vi "Car Wash.vi"() -> ()   [LabVIEW 2023]
uses:
  Controls/Car Wash Indicators.ctl
  Controls/Wash Options.ctl
  Controls/Queued_Data.ctl
  Controls/State.ctl
  Controls/System_Data.ctl
panel:
  out "error out":errorcluster
  in  "error in":errorcluster
  in  "Start":bool
  out "Elapsed Time":dbl format="%0.2f"
  in  "stop":bool
  out "Wash Entry":bool
  in  "Wash Options":T1
  in  "Car Position Slider":u8(slide) max=3 scale=0.0..4.0
  out "Car Wash Indicators":T2
  # "Car Wash Display"
  # "Entry Console"
  # "Car Position Simulation"
  # "Pre-Soak\nH-P Wash\nL-P Wax\nSpot Free Rinse"
  # "Underbody Wash\nBug Remover"
  # "Tire Shine\nAir Dry"
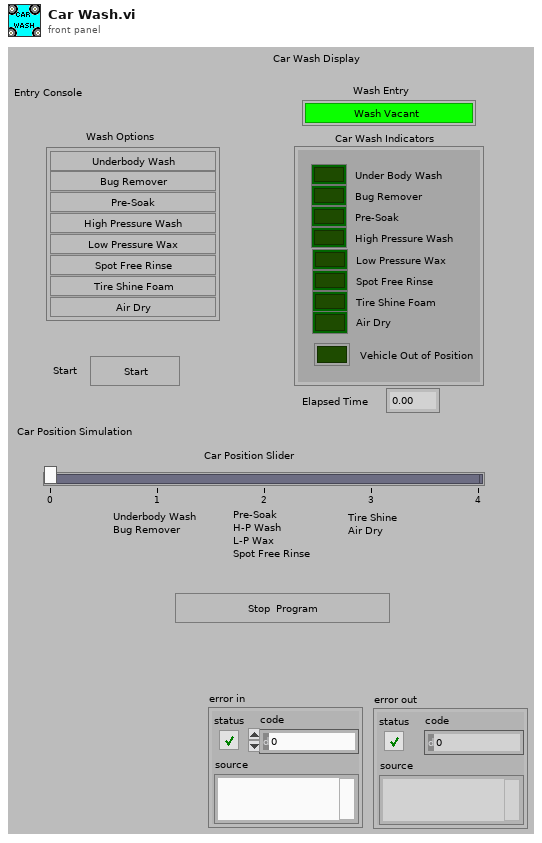
[diagram p1: front panel]
types:
  T1 = typedef "Wash Options.ctl" = cluster{"Underbody Wash":bool, "Bug Remover":bool, "Pre-Soak":bool, "High Pressure Wash":bool, "Low Pressure Wax":bool, "Spot Free Rinse":bool, "Tire Shine Foam":bool, "Air Dry":bool}
  T2 = typedef "Car Wash Indicators.ctl" = cluster{"Under Body Wash":bool, "Bug Remover":bool, "Pre-Soak":bool, "High Pressure Wash":bool, "Low Pressure Wax":bool, "Spot Free Rinse":bool, "Tire Shine Foam":bool, "Air Dry":bool, "Vehicle Out of Position":bool}
  T3 = typedef "State.ctl" = enum16{"Initialize", "Wait for Something", "Step Completed", "Save Wash Options", "Start Process", "Car Position", "Order Steps to follow", "Underbody Wash", "Bug Remover", "Pre-Soak", "High Pressure Wash", "Low Pressure Wax", "Spot Free Rinse", "Tire Shine Foam", "Air Dry", "Vehicle out of position", "Process Complete", "Stop Application"}
  T4 = enum8{"Enabled", "Disabled", "Disabled and Grayed Out"}
  T5 = typedef "System_Data.ctl" = cluster{"Start button":bool, "Wash Options":T1, "Enabled Steps Index":i32[], "Enabled Steps ":T3[], "Index Current Step":i32, "Car Position":u8, "Step Time":dbl[], "Timeout":i32}
  T6 = typedef "Queued_Data.ctl" = cluster{"State":T3, "Data":variant}
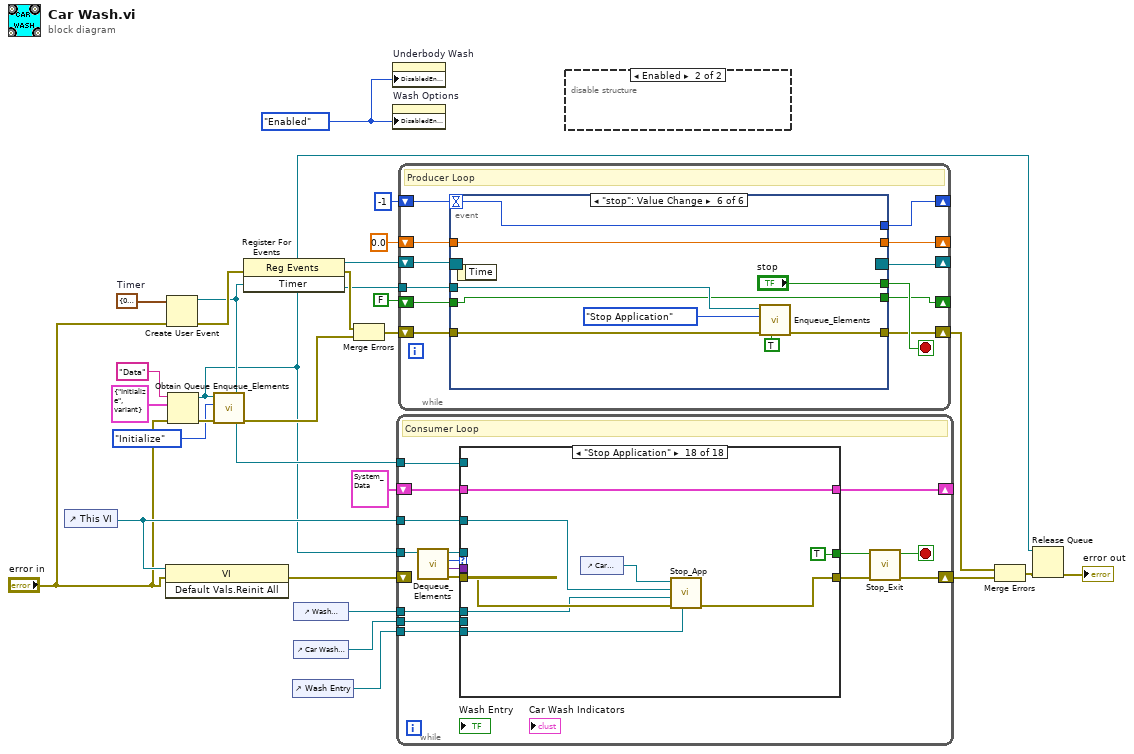
[diagram p0: block diagram]
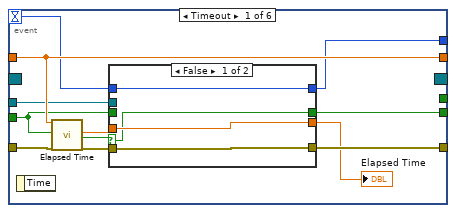
[diagram p2: hidden frame]
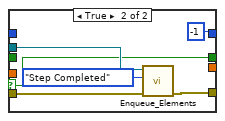
[diagram p3: hidden frame]
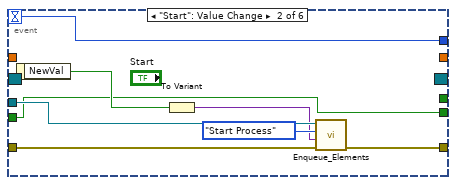
[diagram p4: hidden frame]
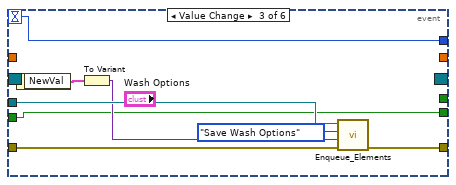
[diagram p5: hidden frame]
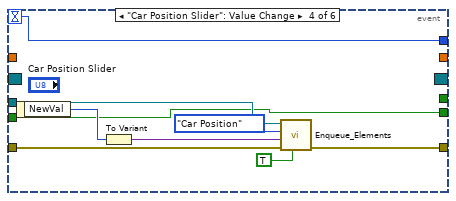
[diagram p6: hidden frame]
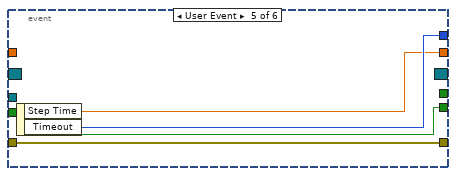
[diagram p7: hidden frame]
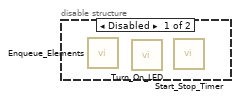
[diagram p8: hidden frame]
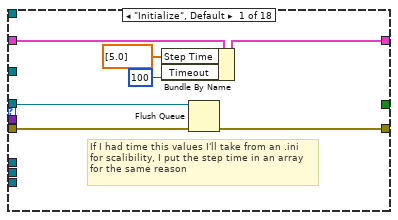
[diagram p9: hidden frame]
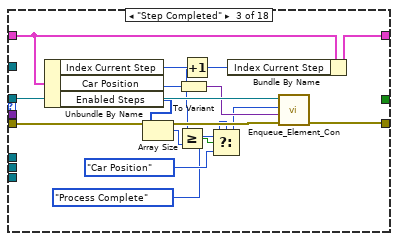
[diagram p11: hidden frame]
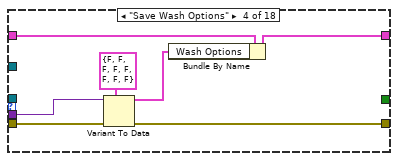
[diagram p12: hidden frame]
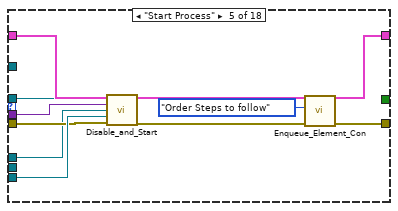
[diagram p13: hidden frame]
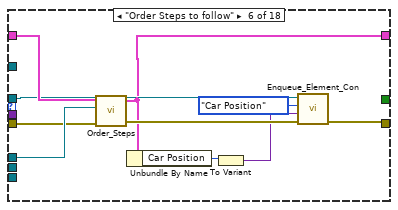
[diagram p14: hidden frame]
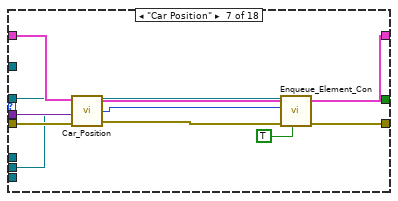
[diagram p15: hidden frame]
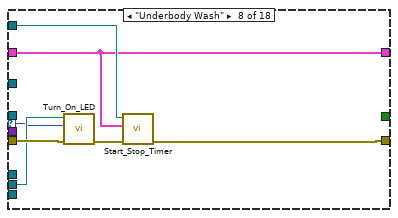
[diagram p16: hidden frame]
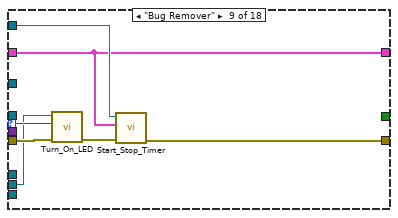
[diagram p17: hidden frame]
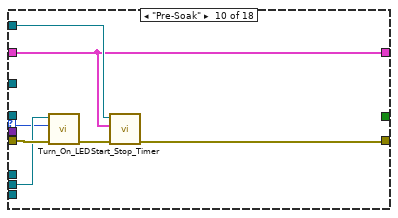
[diagram p18: hidden frame]
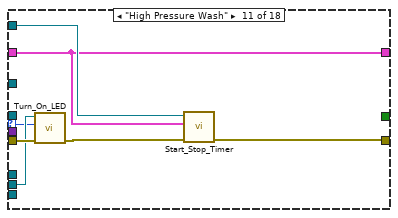
[diagram p19: hidden frame]
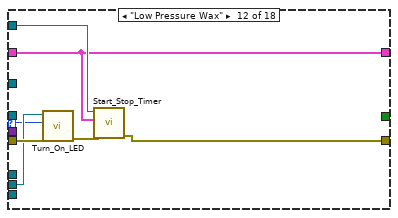
[diagram p20: hidden frame]
diagram:
  w8 = cluster{"Step Time":dbl, "Timeout":i32} {"Step Time"=0.0, "Timeout"=0}  # Timer
  w19 = T4."Enabled" ("Disabled")
  n1 = control-ref of="This VI"() -> (w18:refnum<vi>)
  n2 = invoke class="VI" method="Default Vals.Reinit All"(reference=w18, error in="error in") -> (error out=w17:errorcluster)  [unwired: 1 in, 2 out]
  n3 = Create User Event(user event datatype=w8, error in="error in") -> (user event=w10:refnum<user-event>, error out=w12:errorcluster)
  n4 = Obtain Queue(name (unnamed)="Data", element data type=T6 {"State"=enum."Initialize", "Data"=variant}, error in (no error)="error in") -> (queue out=w2:refnum<queue>, error out=w5:errorcluster)  [unwired: 2 in, 1 out]
  n5 = call "Enqueue_Elements.vi"("error in (no error)"=w5, "State"=State."Initialize", "Queue in"=w2) -> ("error out"=w4:errorcluster)  [unwired: 8 in]
  n6 = register-events(error in=w12, w10) -> (reference out=w11:refnum<event-registration>, error out=w13:errorcluster)  [unwired: 1 in]
  n7 = control-ref of="Wash Entry"() -> (w21:refnum<vi>)
  n8 = control-ref of="Wash Options"() -> (w20:refnum<vi>)
  n9 = control-ref of="Car Wash Indicators"() -> (w22:refnum<vi>)
  n10 = Merge Errors(w13, w4) -> (w15:errorcluster)
  n11 = property on="Underbody Wash" class="Bool (strict)"("DisabledEnum"=w19) -> ()  [unwired: 2 in, 2 out]
  n12 = property on="Wash Options" class="Clust (strict)"("DisabledEnum"=w19) -> ()  [unwired: 2 in, 2 out]
  n13 = while {
    shift-right: [w41] -> w26
    shift-left: w17 -> [_]
    tunnel: w2 -> [w39]
    shift-right: [w36] -> _
    shift-left: T5 {"Start button"=FALSE, "Wash Options"={"Underbody Wash"=FALSE, "Bug Remover"=FALSE, "Pre-Soak"=FALSE, "High Pressure Wash"=FALSE, "Low Pressure Wax"=FALSE, "Spot Free Rinse"=FALSE, "Tire Shine Foam"=FALSE, "Air Dry"=FALSE}, "Enabled Steps Index"=[], "Enabled Steps "=[], "Index Current Step"=0, "Car Position"=0, "Step Time"=[], "Timeout"=0} -> [w37]
    tunnel: w20 -> [w34]
    tunnel: w22 -> [w30]
    tunnel: w21 -> [w33]
    tunnel: w18 -> [w32]
    tunnel: w10 -> [w28]
    stop <- w43 stop-if-true
    # "Consumer Loop"
    n14 = call "Dequeue_Elements.vi"("Queue in"=w39) -> ("error out"=w40:errorcluster, "Data"=w38:variant, "State"=w29:T3, "queue out"=w35:refnum<queue>)  [unwired: 3 in]
    n15 = case shown="\"Stop Application\"" w29 {
      selector: w29 -> [_ _ _ _ _ _ _ w109 w118 w123 w130 w137 w144 w151 w158 _ _ _]
      tunnel: w40 -> [w50 w52 w64 w74 w77 w92 w104 w111 w117 w125 w132 w139 w146 w153 w160 w170 w172 w179]
      tunnel: [w45 w52 w63 w72 w75 w90 w100 w107 w114 w121 w128 w135 w142 w148 w156 w166 w173 w181] -> w42
      tunnel: w38 -> [_ _ _ w71 w83 _ w102 _ _ _ _ _ _ _ _ _ _ _]
      tunnel: w37 -> [w49 w51 w67 w73 w84 w94 w103 w105 w112 w119 w126 w133 w140 w147 w154 w169 w174 w182]
      tunnel: [w48 w51 w65 w69 w82 w87 w101 w105 w112 w119 w126 w133 w140 w147 w154 w169 w174 w182] -> w36
      tunnel: w35 -> [w44 _ w62 _ w80 w89 w98 _ _ _ _ _ _ _ _ _ _ _]
      tunnel: w34 -> [_ _ _ _ w76 w93 _ _ _ _ _ _ _ _ _ _ _ w178]
      tunnel: w30 -> [_ _ _ _ _ _ w95 w110 w116 w124 w131 w138 w145 w152 w159 w167 _ _]
      tunnel: w33 -> [_ _ _ _ w78 _ _ _ _ _ _ _ _ _ _ _ _ w176]
      tunnel: w32 -> [_ _ _ _ _ _ _ _ _ _ _ _ _ _ _ _ w171 w180]
      tunnel: [_ _ _ _ _ _ _ _ _ _ _ _ _ _ _ _ _ TRUE] -> w31
      tunnel: w28 -> [_ _ _ _ _ _ _ w106 w113 w120 w127 w134 w141 w149 w155 _ _ _]
      frame "Initialize", Default {
        # "If I had time this values I'll take from an .ini\nfor scalibility, I put the step time in an array\nfor the same reason"
        n16 = Bundle By Name(cluster=w49, "Step Time"=dbl[] [5.0], "Timeout"=100) -> (w48:T5)
        n17 = Flush Queue(queue=w44, error in (no error)=w50) -> (error out=w45:errorcluster)  [unwired: 2 out]
      }
      frame "Wait for Something" {
      }
      frame "Step Completed" {
        n18 = Unbundle By Name(w67) -> ("Index Current Step"=w66:i32, "Car Position"=w61:u8, "Enabled Steps"=w58:T3[])
        n19 = Array Size(array=w58) -> (size(s)=w57:i32)
        n20 = To Variant(anything=w61) -> (Variant=w60:variant)
        n21 = Increment(x=w66) -> (x+1=w59:i32)
        n22 = Greater Or Equal?(x=w59, y=w57) -> (x >= y?=w56:bool)
        n23 = Select(t=State."Process Complete" ("State"), s=w56, f=State."Car Position" ("State")) -> (s? t:f=w54:T3)
        n24 = Bundle By Name(cluster=w67, "Index Current Step"=w59) -> (w65:T5)
        n25 = call "Enqueue_Element_Con.vi"("error in (no error)"=w64, "Data"=w60, "State"=w54, "Queue in"=w62) -> ("error out"=w63:errorcluster)  [unwired: 7 in]
      }
      frame "Save Wash Options" {
        n26 = Variant To Data(error in=w74, type=T1 {"Underbody Wash"=FALSE, "Bug Remover"=FALSE, "Pre-Soak"=FALSE, "High Pressure Wash"=FALSE, "Low Pressure Wax"=FALSE, "Spot Free Rinse"=FALSE, "Tire Shine Foam"=FALSE, "Air Dry"=FALSE} ("Wash Options"), Variant=w71) -> (data=w68:T1, error out=w72:errorcluster)
        n27 = Bundle By Name(cluster=w73, "Wash Options"=w68) -> (w69:T5)
      }
      frame "Start Process" {
        n28 = call "Disable_and_Start.vi"("System data in"=w84, "Data"=w83, "Wash Options In"=w76, "Wash Entry"=w78, "error in (no error)"=w77) -> ("System data out"=w82:T5, "error out"=w81:errorcluster)  [unwired: 9 in]
        n29 = call "Enqueue_Element_Con.vi"("error in (no error)"=w81, "State"=State."Order Steps to follow", "Queue in"=w80) -> ("error out"=w75:errorcluster)  [unwired: 8 in]
      }
      frame "Order Steps to follow" {
        n30 = call "Order_Steps.vi"("System data"=w94, "Wash Options"=w93, "error in (no error)"=w92) -> ("System data out"=w87:T5, "error out"=w91:errorcluster)  [unwired: 3 in]
        n31 = Unbundle By Name(w87) -> ("Car Position"=w86:u8)
        n32 = To Variant(anything=w86) -> (Variant=w85:variant)
        n33 = call "Enqueue_Element_Con.vi"("error in (no error)"=w91, "Data"=w85, "State"=State."Car Position", "Queue in"=w89) -> ("error out"=w90:errorcluster)  [unwired: 7 in]
      }
      frame "Car Position" {
        n34 = call "Car_Position.vi"("error in (no error)"=w104, "Car Wash Indicators"=w95, "Data"=w102, "System data in"=w103) -> ("error out"=w99:errorcluster, "State"=w97:T3, "System data out"=w101:T5)
        n35 = call "Enqueue_Element_Con.vi"("Prioritize?"=TRUE, "error in (no error)"=w99, "State"=w97, "Queue in"=w98) -> ("error out"=w100:errorcluster)  [unwired: 7 in]
      }
      frame "Underbody Wash" {
        n36 = call "Turn_On_LED.vi"("error in (no error)"=w111, "State"=w109, "Car Wash Indicators"=w110) -> ("error out"=w108:errorcluster)  [unwired: 8 in]
        n37 = call "Start_Stop_Timer.vi"("error in (no error)"=w108, "System data"=w105, "User Event in"=w106) -> ("error out"=w107:errorcluster)  [unwired: 8 in]
      }
      frame "Bug Remover" {
        n38 = call "Turn_On_LED.vi"("error in (no error)"=w117, "State"=w118, "Car Wash Indicators"=w116) -> ("error out"=w115:errorcluster)  [unwired: 8 in]
        n39 = call "Start_Stop_Timer.vi"("error in (no error)"=w115, "System data"=w112, "User Event in"=w113) -> ("error out"=w114:errorcluster)  [unwired: 8 in]
      }
      frame "Pre-Soak" {
        n40 = call "Turn_On_LED.vi"("error in (no error)"=w125, "State"=w123, "Car Wash Indicators"=w124) -> ("error out"=w122:errorcluster)  [unwired: 8 in]
        n41 = call "Start_Stop_Timer.vi"("error in (no error)"=w122, "System data"=w119, "User Event in"=w120) -> ("error out"=w121:errorcluster)  [unwired: 8 in]
      }
      frame "High Pressure Wash" {
        n42 = call "Turn_On_LED.vi"("error in (no error)"=w132, "State"=w130, "Car Wash Indicators"=w131) -> ("error out"=w129:errorcluster)  [unwired: 8 in]
        n43 = call "Start_Stop_Timer.vi"("error in (no error)"=w129, "System data"=w126, "User Event in"=w127) -> ("error out"=w128:errorcluster)  [unwired: 8 in]
      }
      frame "Low Pressure Wax" {
        n44 = call "Turn_On_LED.vi"("error in (no error)"=w139, "State"=w137, "Car Wash Indicators"=w138) -> ("error out"=w136:errorcluster)  [unwired: 8 in]
        n45 = call "Start_Stop_Timer.vi"("error in (no error)"=w136, "System data"=w133, "User Event in"=w134) -> ("error out"=w135:errorcluster)  [unwired: 8 in]
      }
      frame "Spot Free Rinse" {
        n46 = call "Turn_On_LED.vi"("error in (no error)"=w146, "State"=w144, "Car Wash Indicators"=w145) -> ("error out"=w143:errorcluster)  [unwired: 8 in]
        n47 = call "Start_Stop_Timer.vi"("error in (no error)"=w143, "System data"=w140, "User Event in"=w141) -> ("error out"=w142:errorcluster)  [unwired: 8 in]
      }
      frame "Tire Shine Foam" {
        n48 = call "Turn_On_LED.vi"("error in (no error)"=w153, "State"=w151, "Car Wash Indicators"=w152) -> ("error out"=w150:errorcluster)  [unwired: 8 in]
        n49 = call "Start_Stop_Timer.vi"("error in (no error)"=w150, "System data"=w147, "User Event in"=w149) -> ("error out"=w148:errorcluster)  [unwired: 8 in]
      }
      frame "Air Dry" {
        n50 = call "Turn_On_LED.vi"("error in (no error)"=w160, "State"=w158, "Car Wash Indicators"=w159) -> ("error out"=w157:errorcluster)  [unwired: 8 in]
        n51 = call "Start_Stop_Timer.vi"("error in (no error)"=w157, "System data"=w154, "User Event in"=w155) -> ("error out"=w156:errorcluster)  [unwired: 8 in]
      }
      frame "Vehicle out of position" {
        w162 = TRUE ("Vehicle Out of Position")
        n52 = property class="Clust (strict)"(reference=w167, error in=w170) -> (reference out=w165:refnum<vi>, error out=w168:errorcluster, "Value"=w164:T2)
        n53 = Not(x=w162) -> (.not. x?=w161:bool)
        n54 = Bundle By Name(cluster=w164, "Vehicle Out of Position"=w162, "Air Dry"=w161, "Tire Shine Foam"=w161, "Spot Free Rinse"=w161, "Low Pressure Wax"=w161, "High Pressure Wash"=w161, "Pre-Soak"=w161, "Bug Remover"=w161, "Under Body Wash"=w161) -> (w163:T2)
        n55 = property class="Clust (strict)"(reference=w165, error in=w168, "Value"=w163) -> (error out=w166:errorcluster)  [unwired: 1 out]
      }
      frame "Process Complete" {
        n56 = invoke class="VI" method="Default Vals.Reinit All"(reference=w171, error in=w172) -> (error out=w173:errorcluster)  [unwired: 1 in, 2 out]
      }
      frame "Stop Application" {
        n57 = control-ref of="Car Position"() -> (w177:refnum<vi>)
        n58 = call "Stop_App.vi"("Wash Entry"=w176, "error in (no error)"=w179, "Wash Options"=w178, "This VI"=w180, "Car Position"=w177) -> ("error out"=w181:errorcluster)  [unwired: 6 in]
      }
    }
    n59 = call "Stop_Exit.vi"("error in (no error)"=w42, "STOP button"=w31) -> ("error out"=w41:errorcluster, "Exit While"=w43:bool)  [unwired: 8 in]
  }
  n60 = while {
    tunnel: w2 -> [w194]
    shift-right: [w191] -> w14
    shift-left: w15 -> [w193]
    shift-right: [w189] -> _
    shift-left: w11 -> [w190]
    shift-right: [w187] -> _
    shift-left: -1 -> [w188]
    shift-right: [w185] -> _
    shift-left: 0.0 -> [w186]
    shift-right: [w183] -> _
    shift-left: FALSE -> [w184]
    stop <- w192 stop-if-true
    # "Producer Loop"
    n61 = event shown="[5] \"stop\": Value Change" {
      selector: w190 -> [_ _ _ _ _ _]
      dyn-events: [_ _ _ _ _ _] -> w189
      timeout: w188 -> [w202 w218 w226 w234 _ w248]
      tunnel: w194 -> [w197 w224 w230 w241 _ w253]
      tunnel: w193 -> [w206 w223 w231 w237 w245 w251]
      tunnel: [w200 w222 w232 w239 w245 w254] -> w191
      tunnel: [_ _ _ _ _ "stop"] -> w192
      tunnel: [w203 w218 w226 w234 w244 w248] -> w187
      tunnel: w186 -> [w205 _ _ _ _ w247]
      tunnel: [w205 _ _ _ w243 w247] -> w185
      tunnel: w184 -> [w196 w217 w225 w233 w242 w246]
      tunnel: [w195 w217 w225 w233 w242 w246] -> w183
      event Timeout {
        n62 = event-data() -> ()  [unwired: 1 in, 1 out]
        n63 = call "Elapsed Time"("Time Target (s)"=w205, "Reset"=w196, "error in (no error)"=w206) -> ("Elapsed Time (s)"=w198:dbl, "Time has Elapsed"=w204:bool, "error out"=w201:errorcluster)  [unwired: 9 in, 5 out]
        n64 = case shown="False" w204 {
          selector: w204 -> [w207 w211]
          tunnel: [w210 -1 ("t")] -> w203
          tunnel: w202 -> [w210 _]
          tunnel: w198 -> [w208 _]
          tunnel: w201 -> [w209 w214]
          tunnel: [w209 w215] -> w200
          tunnel: [w208 _] -> w199
          tunnel: w197 -> [_ w213]
          tunnel: w196 -> [_ _]
          tunnel: [w207 w211] -> w195
          frame False {
          }
          frame True {
            n65 = call "Enqueue_Elements.vi"("error in (no error)"=w214, "State"=State."Step Completed", "Queue in"=w213) -> ("error out"=w215:errorcluster)  [unwired: 8 in]
          }
        }
        "Elapsed Time" <- w199
      }
      event "Start": Value Change {
        n66 = event-data() -> ("NewVal"=w220:bool)  [unwired: 1 in]
        n67 = To Variant(anything=w220) -> (Variant=w219:variant)
        n68 = call "Enqueue_Elements.vi"("error in (no error)"=w223, "Data"=w219, "State"=State."Start Process", "Queue in"=w224) -> ("error out"=w222:errorcluster)  [unwired: 7 in]
      }
      event Value Change {
        n69 = event-data() -> ("NewVal"=w229:T1)  [unwired: 1 in]
        n70 = To Variant(anything=w229) -> (Variant=w227:variant)
        n71 = call "Enqueue_Elements.vi"("error in (no error)"=w231, "Data"=w227, "State"=State."Save Wash Options", "Queue in"=w230) -> ("error out"=w232:errorcluster)  [unwired: 7 in]
      }
      event "Car Position Slider": Value Change {
        n72 = event-data() -> ("NewVal"=w240:u8)  [unwired: 1 in]
        n73 = To Variant(anything=w240) -> (Variant=w236:variant)
        n74 = call "Enqueue_Elements.vi"("Prioritize?"=TRUE, "error in (no error)"=w237, "Data"=w236, "State"=State."Car Position", "Queue in"=w241) -> ("error out"=w239:errorcluster)  [unwired: 6 in]
      }
      event User Event {
        n75 = event-data() -> ("Step Time"=w243:dbl, "Timeout"=w244:i32)  [unwired: 1 in]
      }
      event "stop": Value Change {
        n76 = event-data() -> ()  [unwired: 1 in, 1 out]
        n77 = call "Enqueue_Elements.vi"("Prioritize?"=TRUE, "error in (no error)"=w251, "State"=State."Stop Application", "Queue in"=w253) -> ("error out"=w254:errorcluster)  [unwired: 7 in]
      }
    }
  }
  n78 = disable-structure shown="Enabled" {
    frame Disabled {
      n79 = call "Enqueue_Elements.vi"() -> ()  [unwired: 11 in, 1 out]
      n80 = call "Turn_On_LED.vi"() -> ()  [unwired: 11 in, 1 out]
      n81 = call "Start_Stop_Timer.vi"() -> ()  [unwired: 11 in, 1 out]
    }
    frame Enabled {
    }
  }
  n82 = Merge Errors(w14, w26) -> (w16:errorcluster)
  n83 = Release Queue(queue=w2, error in (no error)=w16) -> (error out=→"error out":errorcluster)  [unwired: 1 in, 2 out]
